vi "LEP_RV_ConfigureUVProject.vi"(6 "Config":T1 {"Constant Deallocation" items=["Out of Scope", "VI End", "Application End"]; "Constant Allocation" items=["First Use", "Containing Loop", "VI Initialization", "Application Initialization"]; "Target serial port" items=["0", "1", "2", "3"]; "Console output" items=["Processor status window", "Serial port"]; "Optimization" items=["Level 0 (-O0)", "Level 1 (-O1)", "Level 2 (-O2)", "Level 3 (-O3)"]; "Mode" items=["ARM-Mode", "Thumb-Mode"]; "Debug Options" items=["Use ULINK Debugger", "Use Simulator"]; "Debug Mode" items=["Instrumented (serial port)", "Instrumented (TCP/IP)", "Non-instrumented (JTAG/USB)"]}, 8 "error in (no error)":errorcluster, 10 "uVision Project":path, 11 "Target":string) -> (0 "error out":errorcluster)   [LabVIEW 2011]
doc: "Runs the embedded application on a console located in the <B>Build Path</B> directory ."
uses:
  LEP_RV_Config.ctl
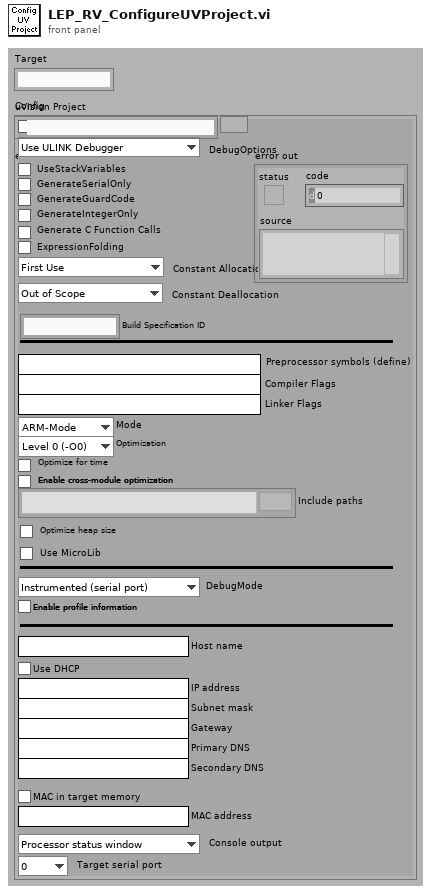
[diagram p1: front panel]
types:
  T1 = typedef "LEP_RV_Config.ctl" = cluster{"Enable debugging":bool, "Debug Options":u16, "Use stack variables":bool, "Generate serial only":bool, "Generate guard code":bool, "Generate Integer Only":bool, "Generate C Function Calls":bool, "ExpressionFolding":bool, "Constant Allocation":u16, "Constant Deallocation":u16, "Build Specification ID":string, "Preprocessor symbols (define)":string, "Compiler Flags":string, "Linker Flags":string, "Mode":u16, "Optimization":u16, "Optimize for time":bool, "Enable cross-module optimization":bool, "Include paths":path[], "Optimize heap size":bool, "Use MicroLib":bool, "Debug Mode":u16, "Enable profile information":bool, "Host name":string, "Use DHCP":bool, "IP address":string, "Subnet mask":string, "Gateway":string, "Primary DNS":string, "Secondary DNS":string, "MAC in target memory":bool, "MAC address":string, "Console output":u16, "Target serial port":u16}
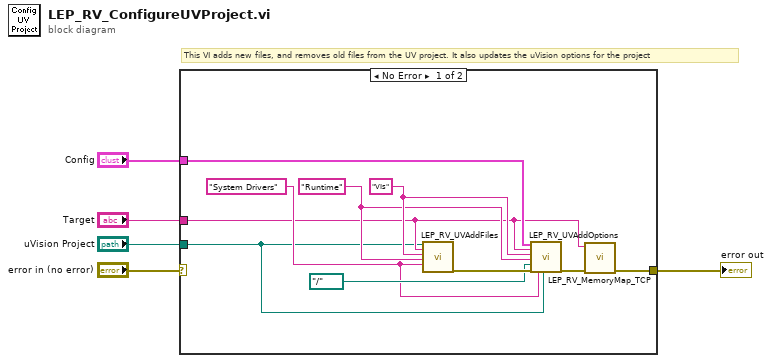
[diagram p0: block diagram]
diagram:
  # "This VI adds new files, and removes old files from the UV project. It also updates the uVision options for the project"
  n1 = case shown="No Error" "error in (no error)" {
    selector: "error in (no error)" -> [_ w16]
    tunnel: [w8 w16] -> w4
    tunnel: "Target" -> [w7 _]
    tunnel: "Config" -> [w14 _]
    tunnel: "uVision Project" -> [w6 _]
    frame No Error {
      w10 = "System Drivers" ("LV Runtime Group Name")
      w12 = "Runtime" ("LV Runtime Group Name")
      w13 = "VIs" ("VI Group Name")
      n2 = call "LEP_RV_UVAddFiles.vi"("uVision Project"=w6, "Target"=w7, "VI Group Name"=w13, "LV Runtime Group Name"=w12, "Driver Group Name"=w10) -> ("error out"=w15:errorcluster)  [unwired: 1 in, 13 out]
      n3 = call "LEP_RV_UVAddOptions.vi"("Config"=w14, "Target"=w7, "VI Group Name"=w13, "LV Runtime Group Name"=w12, "Path to VI Files"=path "../..", "error in (no error)"=w15, "Drivers Group Name"=w10, "uVision Project"=w6) -> ("error out"=w9:errorcluster)  [unwired: 11 out]
      n4 = call "LEP_RV_MemoryMap_TCP.vi"("error in (no error)"=w9, "Target"=w7) -> ("error out"=w8:errorcluster)  [unwired: 9 out]
    }
    frame Error {
    }
  }
  "error out" <- w4
